vi "Receive BBOX (SubVI).vi"() -> (3 "BBox Array":u64[](array[numeric]))   [LabVIEW 2015]
uses:
  <vilib>/rvi/interface/RandomDataEmulation/niFpgaRandomDataHandleErrors.vi
  <vilib>/rvi/DataTransferAndStorage/Container/XNode/niFpgaContainer.xnode
  <vilib>/rvi/interface/RandomDataEmulation/nirviRandomDataFpgaReadWriteTemplate.vi
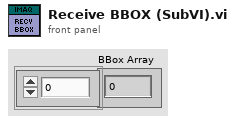
[diagram p1: front panel]
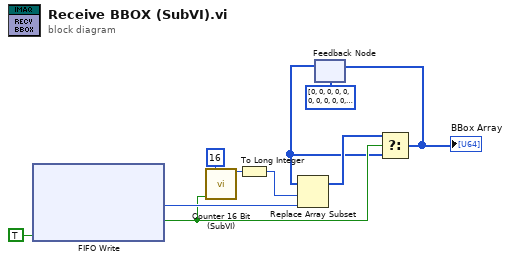
[diagram p0: block diagram]
diagram:
  n1 = xnode ("FIFO Write")("Ready for Output"=TRUE) -> ("Element"=w10:u64, "Output Valid"=w2:bool)  [unwired: 1 in, 1 out]
  n2 = call "Counter 16 Bit (SubVI).vi"("Max. Count"=u16 16, "Enable"=w2) -> ("Count"=w5:u16)  [unwired: 11 in, 2 out]
  n3 = To Long Integer(number=w5) -> (32bit integer=w4:i32)
  n4 = feedback #1(u64[] [0, 0, 0, 0, 0, 0, 0, 0, 0, 0, 0, 0, 0, 0, 0, 0]) -> (w1:u64[])
  n5 = Replace Array Subset(array=w1, new element=w10, index=w4) -> (w9:u64[])
  n6 = Select(t=w9, s=w2, f=w1) -> (s? t:f=w3:u64[])
  "BBox Array" <- w3
  n7 = feedback-in #1(w3) -> ()
